vi "MDrive_Set_Parameter.vi"(4 "Device Name":string, 6 "Mdrive Mode":T1=enum."Party Mode", 8 "error in":errorcluster, 9 "Parameter Setpoint":string, 10 "Set Parameter":T2, 11 "VISA IN":refnum<visa-resource-name>) -> (0 "error out":errorcluster, 1 "read buffer":string, 3 "VISA OUT":refnum<visa-resource-name>)   [LabVIEW 2015]
uses:
  Set Parameter.ctl
  MDrive Mode.ctl
  Stream/LP Globals.vi
panel:
  out "Command out":string
  # "(Only in party mode)"
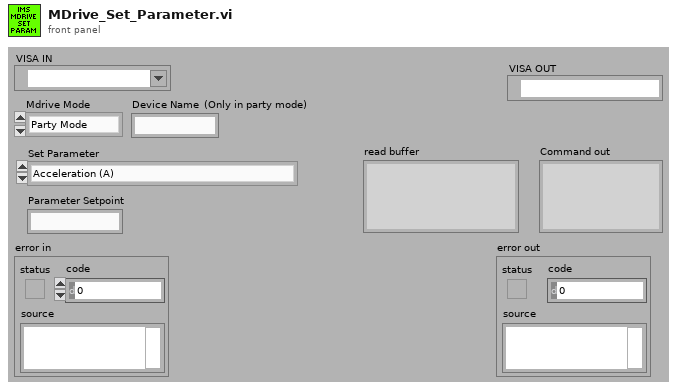
[diagram p1: front panel]
types:
  T1 = typedef "MDrive Mode.ctl" = enum16{"Normal Mode", "Party Mode"}
  T2 = typedef "Set Parameter.ctl" = enum16{"Acceleration (A)", "Baud Rate (BD)", "Counter 1 (C1)", "Counter 2 (C2)", "Control C Software Reset (CE)", "Check Sum Enable (CK)", "Clock Mode (CM)", "Clock Mode Ratio (CR)", "Clock Mode Out Step Width (CW)", "Deceleration (D)", "Digital Filtering, Input 1 (D1)", "Digital Filtering, Input 2 (D2)", "Digital Filtering, Input 3 (D3)", "Digital Filtering, Input 4 (D4)", "Digital Filtering, Input 5 (D5)", "Digital Filtering, Input 9 (D9)", "Digital Filtering, Input 10 (D10)", "Digital Filtering, Input 11 (D11)", "Digital Filtering, Input 12 (D12)", "Deadband (DB)", "Decrement Variable (DC)", "Enable/Disable Drive (DE)", "Device Name (DN)", "End Program Execution (E)", "Encoder Function Enable (EE)", "Encoder Lines (EL)", "Echo Mode (EM)", "Error Clear (ER)", "Escape (ES)", "Execute Program at Address (EX)", "Factory Default (FD)", "Hold (H)", "Hold Current (HC)", "Hold Current Encoder Index (HI)", "Home to Home Switch (HM)", "Home to Delay Time (HT)", "Increment Variable (IC)", "Initialize Parameters to NVM (IP)", "Input into Variable (IV)", "Jog Enable (JE)", "Limit Stop Mode (LM)", "Move Absolute (MA)", "Move Relative (MR)", "MicroStepping Select (MS)", "Motor Settling Delay Time (MT)", "Output 1 (O1)", "Output 2 (O2)", "Output 3 (O3)", "Output 4 (O4)", "Output 9 (O9)", "Output 10 (O10)", "Output 11 (O11)", "Output 12 (O12)", "Output High Byte (9-12) (OH)", "Output Low Byte (1-4) (OL)", "Output Total (1-4 and 9-12) (OT)", "Position (P)", "Position Maintenance (PM)", "Party Mode (PY)", "Register 1 (R1)", "Register 2 (R2)", "Register 3 (R3)", "Register 4 (R4)", "Run Current (RC)", "Stall Factor (SF)", "Slew (SL)", "Stall Mode Set (SM)", "Upgrade Firmware (UG)", "Velocity Initial (VI)", "Velocity Maximum (VM)", "Set Input #1 as Home (S1)", "Save (S)", "Save DN+PY (NameS)", "Active Party Mode (0x0A)", "Set Input #1 (S1) as Limit- Active Floating", "Set Input #2 (S2) as Limit+ Active Floating", "Set Input #1 as Home (S1) Active Floating", "Set Input #1 as Home (S2) Active Floating", "Set Input #1 (S1) as Limit+ Active Floating", "Set Input #2 (S2) as Limit- Active Floating", "Hybrid Mode (AS)"}
  T3 = typedef "Semaphore RefNum" = refnum<k1>
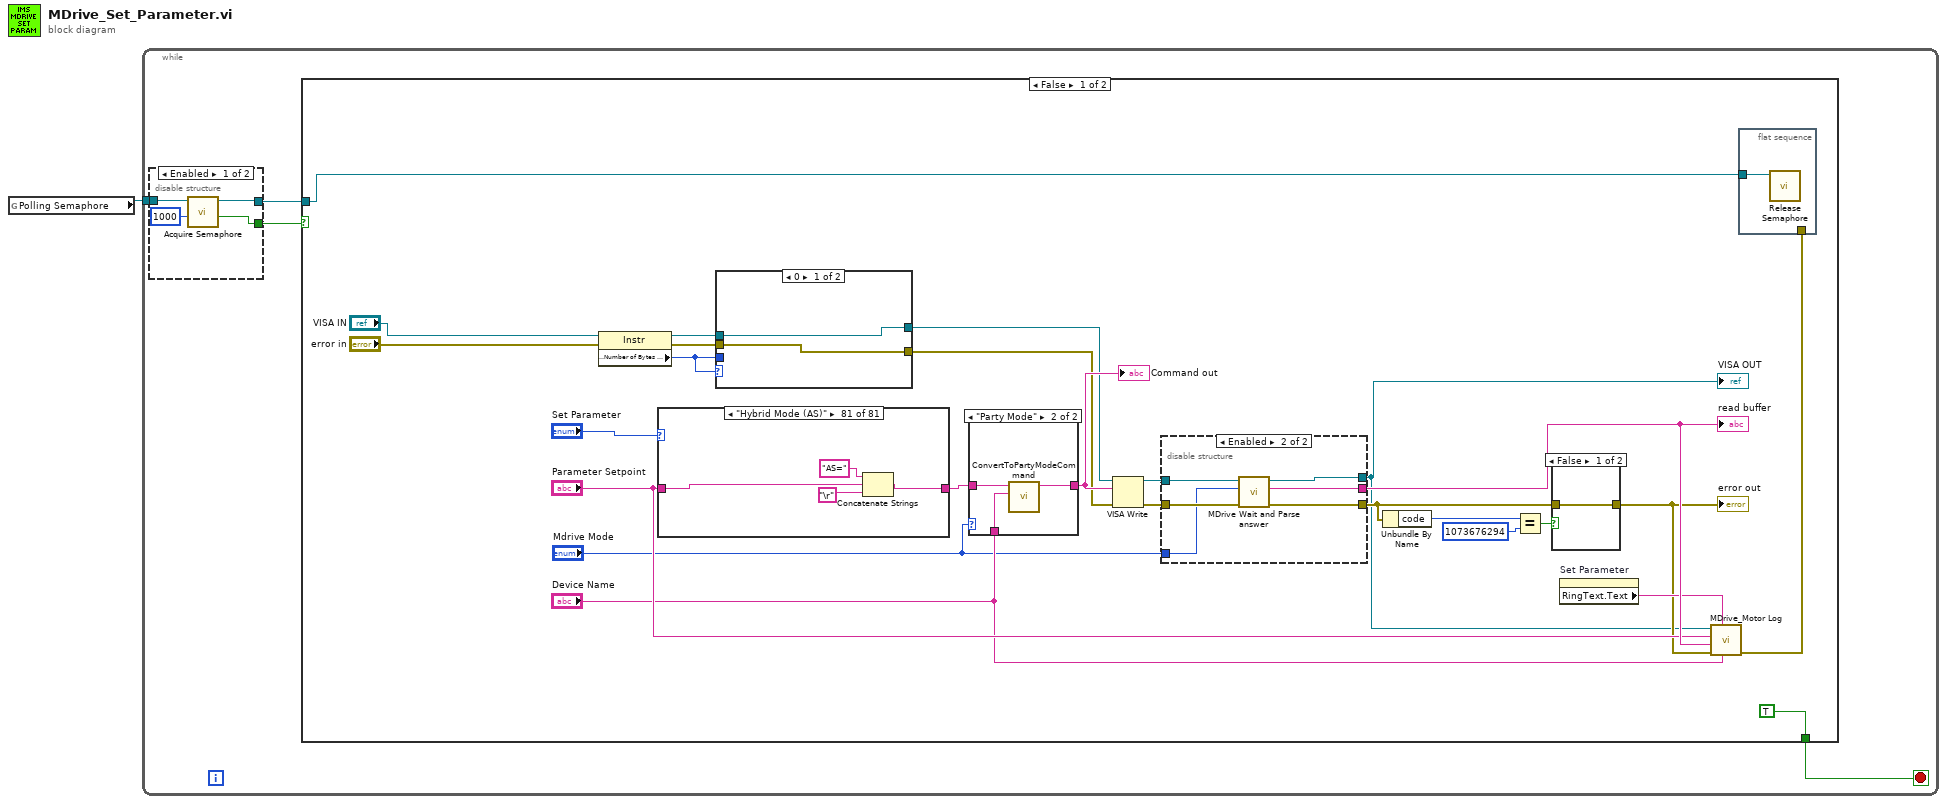
[diagram p0: block diagram]
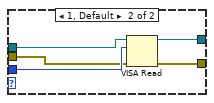
[diagram p3: hidden frame]
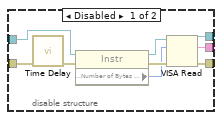
[diagram p4: hidden frame]
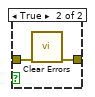
[diagram p6: hidden frame]
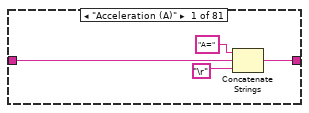
[diagram p7: hidden frame]
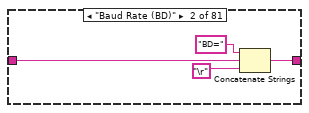
[diagram p8: hidden frame]
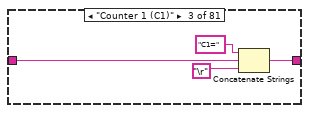
[diagram p9: hidden frame]
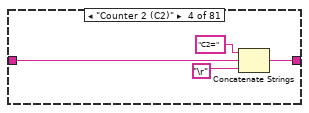
[diagram p10: hidden frame]
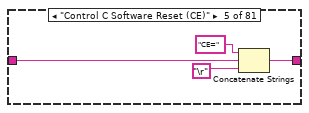
[diagram p11: hidden frame]
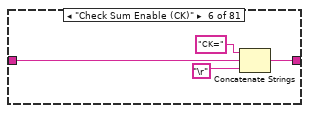
[diagram p12: hidden frame]
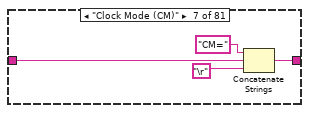
[diagram p13: hidden frame]
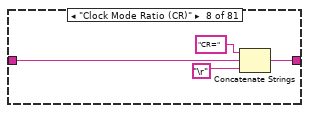
[diagram p14: hidden frame]
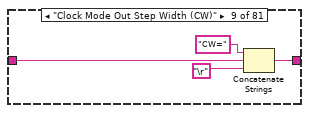
[diagram p15: hidden frame]
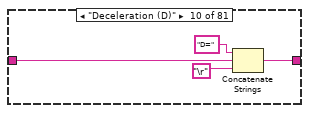
[diagram p16: hidden frame]
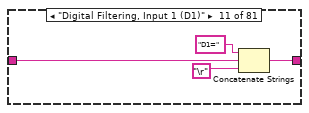
[diagram p17: hidden frame]
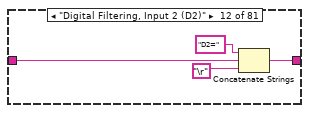
[diagram p18: hidden frame]
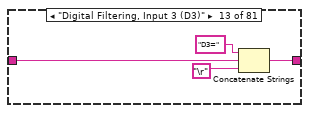
[diagram p19: hidden frame]
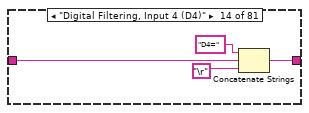
[diagram p20: hidden frame]
diagram:
  n1 = global read "LP Globals.vi" "Polling Semaphore"() -> (w1:T3)
  n2 = while {
    tunnel: w1 -> [w5]
    stop <- w3 stop-if-true
    n3 = disable-structure shown="Enabled" {
      disable-tunnel: w5 -> [w9 _]
      disable-tunnel: [w8 _] -> w4
      disable-tunnel: [w6 _] -> w2
      frame Enabled {
        n4 = call <vilib>:"Acquire Semaphore.vi"("ms timeout (-1)"=1000, "semaphore"=w9) -> ("timed out"=w6:bool, "semaphore out"=w8:T3)  [unwired: 3 in, 1 out]
      }
      frame Disabled {
      }
    }
    n5 = case shown="False" w2 {
      tunnel: w4 -> [w11 _]
      tunnel: [TRUE _] -> w3
      frame False {
        n6 = property class="Instr"(reference="VISA IN", error in="error in") -> (reference out=w13:refnum<visa-resource-name>, error out=w14:errorcluster, "Serial Settings:Number of Bytes at Serial Port"=w12:u32)
        n7 = case shown="\"Hybrid Mode (AS)\"" "Set Parameter" {
          tunnel: "Parameter Setpoint" -> [w67 w70 w75 w79 w82 w86 w90 w94 w98 w102 w106 w110 w114 w118 w122 w126 w130 w134 w138 w142 w146 w150 w155 w159 w163 w167 _ _ w178 w182 w186 _ w193 w197 w201 w205 w209 w213 w217 w221 w225 w229 w233 w237 w241 w245 w249 w253 w257 w261 w265 w269 w273 w277 w281 w285 w289 w293 w297 w301 _ w307 w310 w314 w318 w322 w326 w330 w334 w338 w342 w347 w350 _ _ _ _ _ _ _ w382]
          tunnel: [w66 w71 w74 w78 w83 w87 w91 w95 w99 w103 w107 w111 w115 w119 w123 w127 w131 w135 w139 w143 w147 w151 w157 w160 w164 w168 w172 w176 w179 w183 w187 w190 w194 w198 w202 w206 w210 w214 w218 w222 w226 w230 w234 w238 w242 w246 w250 w254 w258 w262 w266 w270 w274 w278 w282 w286 w290 w294 w298 w302 "\n" w306 w311 w315 w319 w323 w327 w331 w335 w339 w343 w346 w351 w355 w359 w363 w367 w371 w375 w379 w383] -> w30
          frame "Acceleration (A)" {
            n8 = Concatenate Strings("A=" ("string"), w67, "\r") -> (w66:string)
          }
          frame "Baud Rate (BD)" {
            n9 = Concatenate Strings("BD=" ("string"), w70, "\r") -> (w71:string)
          }
          frame "Counter 1 (C1)" {
            n10 = Concatenate Strings("C1=" ("string"), w75, "\r") -> (w74:string)
          }
          frame "Counter 2 (C2)" {
            n11 = Concatenate Strings("C2=" ("string"), w79, "\r") -> (w78:string)
          }
          frame "Control C Software Reset (CE)" {
            n12 = Concatenate Strings("CE=" ("string"), w82, "\r") -> (w83:string)
          }
          frame "Check Sum Enable (CK)" {
            n13 = Concatenate Strings("CK=" ("string"), w86, "\r") -> (w87:string)
          }
          frame "Clock Mode (CM)" {
            n14 = Concatenate Strings("CM=" ("string"), w90, "\r") -> (w91:string)
          }
          frame "Clock Mode Ratio (CR)" {
            n15 = Concatenate Strings("CR=" ("string"), w94, "\r") -> (w95:string)
          }
          frame "Clock Mode Out Step Width (CW)" {
            n16 = Concatenate Strings("CW=" ("string"), w98, "\r") -> (w99:string)
          }
          frame "Deceleration (D)" {
            n17 = Concatenate Strings("D=" ("string"), w102, "\r") -> (w103:string)
          }
          frame "Digital Filtering, Input 1 (D1)" {
            n18 = Concatenate Strings("D1=" ("string"), w106, "\r") -> (w107:string)
          }
          frame "Digital Filtering, Input 2 (D2)" {
            n19 = Concatenate Strings("D2=" ("string"), w110, "\r") -> (w111:string)
          }
          frame "Digital Filtering, Input 3 (D3)" {
            n20 = Concatenate Strings("D3=" ("string"), w114, "\r") -> (w115:string)
          }
          frame "Digital Filtering, Input 4 (D4)" {
            n21 = Concatenate Strings("D4=" ("string"), w118, "\r") -> (w119:string)
          }
          frame "Digital Filtering, Input 5 (D5)" {
            n22 = Concatenate Strings("D5=" ("string"), w122, "\r") -> (w123:string)
          }
          frame "Digital Filtering, Input 9 (D9)" {
            n23 = Concatenate Strings("D9=" ("string"), w126, "\r") -> (w127:string)
          }
          frame "Digital Filtering, Input 10 (D10)" {
            n24 = Concatenate Strings("D10=" ("string"), w130, "\r") -> (w131:string)
          }
          frame "Digital Filtering, Input 11 (D11)" {
            n25 = Concatenate Strings("D11=" ("string"), w134, "\r") -> (w135:string)
          }
          frame "Digital Filtering, Input 12 (D12)" {
            n26 = Concatenate Strings("D12=" ("string"), w138, "\r") -> (w139:string)
          }
          frame "Deadband (DB)" {
            n27 = Concatenate Strings("DB=" ("string"), w142, "\r") -> (w143:string)
          }
          frame "Decrement Variable (DC)" {
            n28 = Concatenate Strings("DC=" ("string"), w146, "\r") -> (w147:string)
          }
          frame "Enable/Disable Drive (DE)" {
            n29 = Concatenate Strings("DE=" ("string"), w150, "\r") -> (w151:string)
          }
          frame "Device Name (DN)" {
            w154 = "\""
            n30 = Concatenate Strings("DN=" ("string"), w154, w155, w154, "\r") -> (w157:string)
          }
          frame "End Program Execution (E)" {
            n31 = Concatenate Strings("E=" ("string"), w159, "\r") -> (w160:string)
          }
          frame "Encoder Function Enable (EE)" {
            n32 = Concatenate Strings("EE=" ("string"), w163, "\r") -> (w164:string)
          }
          frame "Echo Mode (EM)" {
            n33 = Concatenate Strings("EM=" ("string"), w167, "\r") -> (w168:string)
          }
          frame "Error Clear (ER)" {
            n34 = Concatenate Strings("ER=" ("string"), "0" ("string"), "\r") -> (w172:string)
          }
          frame "Save (S)" {
            n35 = Concatenate Strings("S" ("string"), "\r") -> (w176:string)
          }
          frame "Save DN+PY (NameS)" {
            n36 = Concatenate Strings(w178, "S" ("string"), "\n") -> (w179:string)
          }
          frame "Escape (ES)" {
            n37 = Concatenate Strings("ES=" ("string"), w182, "\r") -> (w183:string)
          }
          frame "Execute Program at Address (EX)" {
            n38 = Concatenate Strings("EX=" ("string"), w186, "\r") -> (w187:string)
          }
          frame "Factory Default (FD)" {
            n39 = Concatenate Strings("FD" ("string"), "\r") -> (w190:string)
          }
          frame "Hold (H)" {
            n40 = Concatenate Strings("H=" ("string"), w193, "\r") -> (w194:string)
          }
          frame "Hold Current (HC)" {
            n41 = Concatenate Strings("HC=" ("string"), w197, "\r") -> (w198:string)
          }
          frame "Hold Current Encoder Index (HI)" {
            n42 = Concatenate Strings("HI=" ("string"), w201, "\r") -> (w202:string)
          }
          frame "Home to Home Switch (HM)" {
            n43 = Concatenate Strings("HM=" ("string"), w205, "\r") -> (w206:string)
          }
          frame "Home to Delay Time (HT)" {
            n44 = Concatenate Strings("HT=" ("string"), w209, "\r") -> (w210:string)
          }
          frame "Increment Variable (IC)" {
            n45 = Concatenate Strings("IC=" ("string"), w213, "\r") -> (w214:string)
          }
          frame "Initialize Parameters to NVM (IP)" {
            n46 = Concatenate Strings("IP=" ("string"), w217, "\r") -> (w218:string)
          }
          frame "Input into Variable (IV)" {
            n47 = Concatenate Strings("IV=" ("string"), w221, "\r") -> (w222:string)
          }
          frame "Jog Enable (JE)" {
            n48 = Concatenate Strings("JE=" ("string"), w225, "\r") -> (w226:string)
          }
          frame "Limit Stop Mode (LM)" {
            n49 = Concatenate Strings("LM=" ("string"), w229, "\r") -> (w230:string)
          }
          frame "Move Absolute (MA)" {
            n50 = Concatenate Strings("MA=" ("string"), w233, "\r") -> (w234:string)
          }
          frame "Move Relative (MR)" {
            n51 = Concatenate Strings("MR=" ("string"), w237, "\r") -> (w238:string)
          }
          frame "MicroStepping Select (MS)" {
            n52 = Concatenate Strings("MS=" ("string"), w241, "\r") -> (w242:string)
          }
          frame "Motor Settling Delay Time (MT)" {
            n53 = Concatenate Strings("MT=" ("string"), w245, "\r") -> (w246:string)
          }
          frame "Output 1 (O1)" {
            n54 = Concatenate Strings("O1=" ("string"), w249, "\r") -> (w250:string)
          }
          frame "Output 2 (O2)" {
            n55 = Concatenate Strings("O2=" ("string"), w253, "\r") -> (w254:string)
          }
          frame "Output 3 (O3)" {
            n56 = Concatenate Strings("O3=" ("string"), w257, "\r") -> (w258:string)
          }
          frame "Output 4 (O4)" {
            n57 = Concatenate Strings("O4=" ("string"), w261, "\r") -> (w262:string)
          }
          frame "Output 9 (O9)" {
            n58 = Concatenate Strings("O9=" ("string"), w265, "\r") -> (w266:string)
          }
          frame "Output 10 (O10)" {
            n59 = Concatenate Strings("O10=" ("string"), w269, "\r") -> (w270:string)
          }
          frame "Output 11 (O11)" {
            n60 = Concatenate Strings("O11=" ("string"), w273, "\r") -> (w274:string)
          }
          frame "Output 12 (O12)" {
            n61 = Concatenate Strings("O12=" ("string"), w277, "\r") -> (w278:string)
          }
          frame "Output High Byte (9-12) (OH)" {
            n62 = Concatenate Strings("OH=" ("string"), w281, "\r") -> (w282:string)
          }
          frame "Output Low Byte (1-4) (OL)" {
            n63 = Concatenate Strings("OL=" ("string"), w285, "\r") -> (w286:string)
          }
          frame "Output Total (1-4 and 9-12) (OT)" {
            n64 = Concatenate Strings("OT=" ("string"), w289, "\r") -> (w290:string)
          }
          frame "Position (P)" {
            n65 = Concatenate Strings("P=" ("string"), w293, "\r") -> (w294:string)
          }
          frame "Position Maintenance (PM)" {
            n66 = Concatenate Strings("PM=" ("string"), w297, "\r") -> (w298:string)
          }
          frame "Party Mode (PY)" {
            n67 = Concatenate Strings("PY=" ("string"), w301, "\r") -> (w302:string)
          }
          frame "Active Party Mode (0x0A)" {
          }
          frame "Register 1 (R1)" {
            n68 = Concatenate Strings("R1=" ("string"), w307, "\r") -> (w306:string)
          }
          frame "Register 2 (R2)" {
            n69 = Concatenate Strings("R2=" ("string"), w310, "\r") -> (w311:string)
          }
          frame "Register 3 (R3)" {
            n70 = Concatenate Strings("R3=" ("string"), w314, "\r") -> (w315:string)
          }
          frame "Register 4 (R4)" {
            n71 = Concatenate Strings("R4=" ("string"), w318, "\r") -> (w319:string)
          }
          frame "Run Current (RC)" {
            n72 = Concatenate Strings("RC=" ("string"), w322, "\r") -> (w323:string)
          }
          frame "Stall Factor (SF)" {
            n73 = Concatenate Strings("SF=" ("string"), w326, "\r") -> (w327:string)
          }
          frame "Slew (SL)" {
            n74 = Concatenate Strings("SL=" ("string"), w330, "\r") -> (w331:string)
          }
          frame "Stall Mode Set (SM)" {
            n75 = Concatenate Strings("SM=" ("string"), w334, "\r") -> (w335:string)
          }
          frame "Upgrade Firmware (UG)" {
            n76 = Concatenate Strings("UG=" ("string"), w338, "\r") -> (w339:string)
          }
          frame "Velocity Initial (VI)" {
            n77 = Concatenate Strings("VI=" ("string"), w342, "\r") -> (w343:string)
          }
          frame "Velocity Maximum (VM)" {
            n78 = Concatenate Strings("VM=" ("string"), w347, "\r") -> (w346:string)
          }
          frame "Encoder Lines (EL)" {
            n79 = Concatenate Strings("EL=" ("string"), w350, "\r") -> (w351:string)
          }
          frame "Set Input #1 as Home (S1)" {
            # "Active on Low"
            n80 = Concatenate Strings("IS=" ("string"), "1,1,0" ("Parameter Setpoint"), "\r") -> (w355:string)
          }
          frame "Set Input #1 (S1) as Limit- Active Floating" {
            (unwired) "2,1,0" ("Parameter Setpoint")
            # "Active on Floating"
            n81 = Concatenate Strings("IS=" ("string"), "1,3,0" ("Parameter Setpoint"), "\r") -> (w359:string)
          }
          frame "Set Input #2 (S2) as Limit+ Active Floating" {
            (unwired) "2,1,0" ("Parameter Setpoint")
            # "Active on Floating"
            n82 = Concatenate Strings("IS=" ("string"), "2,2,0" ("Parameter Setpoint"), "\r") -> (w363:string)
          }
          frame "Set Input #1 (S1) as Limit+ Active Floating" {
            (unwired) "2,1,0" ("Parameter Setpoint")
            # "Active on Floating"
            n83 = Concatenate Strings("IS=" ("string"), "1,2,0" ("Parameter Setpoint"), "\r") -> (w367:string)
          }
          frame "Set Input #2 (S2) as Limit- Active Floating" {
            (unwired) "2,1,0" ("Parameter Setpoint")
            # "Active on Floating"
            n84 = Concatenate Strings("IS=" ("string"), "2,3,0" ("Parameter Setpoint"), "\r") -> (w371:string)
          }
          frame "Set Input #1 as Home (S1) Active Floating" {
            # "Active on Floating"
            n85 = Concatenate Strings("IS=" ("string"), "1,1,0" ("Parameter Setpoint"), "\r") -> (w375:string)
          }
          frame "Set Input #1 as Home (S2) Active Floating" {
            # "Active on Floating"
            n86 = Concatenate Strings("IS=" ("string"), "2,1,0" ("Parameter Setpoint"), "\r") -> (w379:string)
          }
          frame "Hybrid Mode (AS)" {
            n87 = Concatenate Strings("AS=" ("string"), w382, "\r") -> (w383:string)
          }
        }
        n88 = case shown="0" w12 {
          tunnel: w12 -> [_ w43]
          tunnel: w14 -> [w37 w42]
          tunnel: w13 -> [w38 w41]
          tunnel: [w38 w40] -> w22
          tunnel: [w37 w39] -> w18
          frame 0 {
          }
          frame 1, Default {
            n89 = VISA Read(VISA resource name=w41, byte count=w43, error in (no error)=w42) -> (VISA resource name out=w40:refnum<visa-resource-name>, error out=w39:errorcluster)  [unwired: 2 out]
          }
        }
        n90 = case shown="\"Party Mode\"" "Mdrive Mode" {
          tunnel: "Device Name" -> [_ w62]
          tunnel: w30 -> [w59 w61]
          tunnel: [w59 w60] -> w29
          frame "Normal Mode", Default {
          }
          frame "Party Mode" {
            n91 = call "ConvertToPartyModeCommand.vi"("Device Name"=w62, "Command"=w61) -> ("Command out"=w60:string)  [unwired: 9 in]
          }
        }
        "Command out" <- w29
        n92 = VISA Write(VISA resource name=w22, write buffer=w29, error in (no error)=w18) -> (VISA resource name out=w17:refnum<visa-resource-name>, error out=w35:errorcluster)  [unwired: 1 out]
        n93 = disable-structure shown="Enabled" {
          disable-tunnel: w35 -> [w50 w57]
          disable-tunnel: w17 -> [w49 w58]
          disable-tunnel: [w46 w56] -> w31
          disable-tunnel: [w45 w55] -> w28
          disable-tunnel: [w44 w54] -> w16
          disable-tunnel: "Mdrive Mode" -> [_ w53]
          frame Disabled {
            n94 = call "Time Delay"("error in (no error)"=w50) -> ("error out"=w48:errorcluster)  [unwired: 10 in]
            n95 = property class="Instr"(reference=w49, error in=w48) -> (reference out=w52:refnum<visa-resource-name>, error out=w51:errorcluster, "Serial Settings:Number of Bytes at Serial Port"=w47:u32)
            n96 = VISA Read(VISA resource name=w52, byte count=w47, error in (no error)=w51) -> (VISA resource name out=w44:refnum<visa-resource-name>, read buffer=w45:string, error out=w46:errorcluster)  [unwired: 1 out]
          }
          frame Enabled {
            n97 = call "MDrive Wait and Parse answer.vi"("error in (no error)"=w57, "Mdrive Mode"=w53, "VISA Refnum in"=w58) -> ("error out"=w56:errorcluster, "String"=w55:string, "VISA Refnum out"=w54:refnum<visa-resource-name>)  [unwired: 6 in]
          }
        }
        "VISA OUT" <- w16
        "read buffer" <- w28
        n98 = Unbundle By Name(w31) -> ("code"=w34:i32)
        n99 = Equal?(x=w34, y=1073676294 ("code")) -> (x = y?=w32:bool)
        n100 = case shown="False" w32 {
          tunnel: w31 -> [w63 w65]
          tunnel: [w63 w64] -> w21
          frame False {
          }
          frame True {
            n101 = call <vilib>:"Clear Errors.vi"("error in (no error)"=w65) -> ("error out"=w64:errorcluster)  [unwired: 5 in, 1 out]
          }
        }
        "error out" <- w21
        n102 = property on="Set Parameter" class="Enum (strict)"() -> ("RingText.Text"=w27:string)  [unwired: 2 in, 2 out]
        n103 = call "MDrive_Motor Log.vi"("Motor Name"="Device Name", "Function"=w27, "Error in"=w21, "read buffer"=w28, "Param"="Parameter Setpoint", "COM"=w16) -> ("Error out"=w10:errorcluster)  [unwired: 5 in]
        n104 = flat-sequence {
          tunnel: w11 -> [w36]
          tunnel: w10 -> [_]
          frame #0 {
            n105 = call <vilib>:"Release Semaphore.vi"("semaphore"=w36) -> ()  [unwired: 5 in, 2 out]
          }
        }
      }
      frame True {
      }
    }
  }
